vi "Read.vi"(8 "error in (no error)":errorcluster, 9 "Variant":variant, 11 "UDP in":refnum<class "UDP.lvclass">) -> (0 "error out":errorcluster, 2 "String":string, 3 "UDP out":refnum<class "UDP.lvclass">)   [LabVIEW 2013, in "Protocol Classes.lvlib" / "UDP.lvclass"]
uses:
  UDP.lvclass
  Protocol Parent/Methods/Read Parameter.ctl
  UDP.lvclass/UDP.ctl
  Data Access/Read UDP Ref.vi
  Data Access/Write UDP Ref.vi
  Protocol Parent/Protocol Parent.lvclass
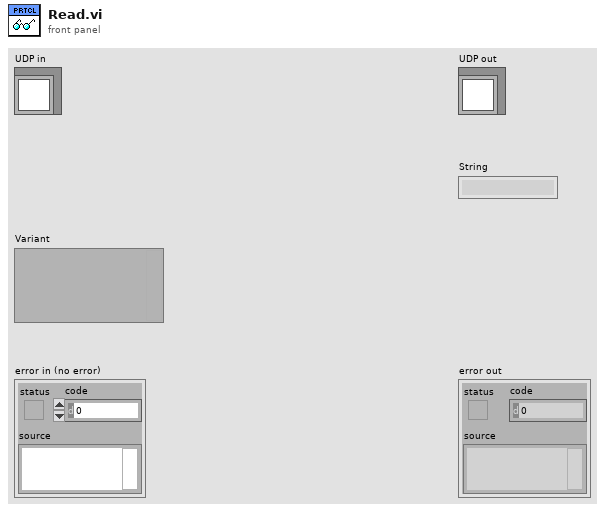
[diagram p1: front panel]
types:
  T1 = typedef "Protocol Classes.lvlib/Protocol Parent.lvclass/Read Parameter.ctl" = cluster{"Wait Type":enum16{"Byte Count", "Wait sec"}, "Wait Value":dbl}
  T2 = enum16{"Standard", "Buffered", "CRLF", "Immediate"}
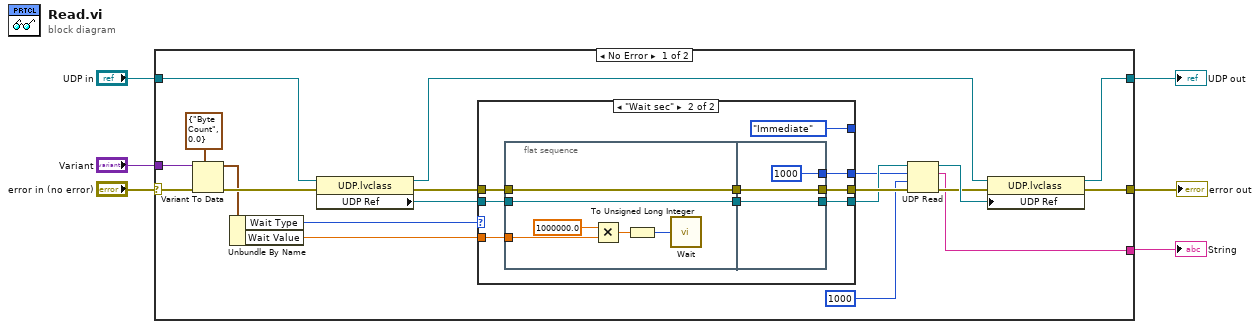
[diagram p0: block diagram]
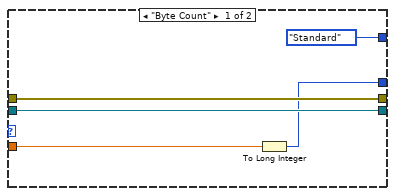
[diagram p2: hidden frame]
diagram:
  n1 = case shown="No Error" "error in (no error)" {
    selector: "error in (no error)" -> [w20 w51]
    tunnel: "UDP in" -> [w26 w50]
    tunnel: [w23 w51] -> w3
    tunnel: [w21 w50] -> w1
    tunnel: "Variant" -> [w18 _]
    tunnel: [w11 _] -> w2
    frame No Error {
      n2 = Variant To Data(error in=w20, type=T1 {"Wait Type"=enum."Byte Count", "Wait Value"=0.0} ("Read Parameter"), Variant=w18) -> (data=w17:T1, error out=w19:errorcluster)
      n3 = Unbundle By Name(w17) -> ("Wait Type"=w13:enum16{"Byte Count", "Wait sec"}, "Wait Value"=w12:dbl)
      n4 = property class="UDP.lvclass"(reference=w26, error in=w19) -> (reference out=w22:refnum<class "UDP.lvclass">, error out=w16:errorcluster, "UDP Ref"=w15:refnum<k16>)
      n5 = case shown="\"Wait sec\"" w13 {
        tunnel: w16 -> [w31 w40]
        tunnel: w15 -> [w29 w39]
        tunnel: [w31 w38] -> w14
        tunnel: [w29 w37] -> w8
        tunnel: [w27 w33] -> w7
        tunnel: w12 -> [w30 w34]
        tunnel: [T2."Standard" ("mode (standard)") T2."Immediate" ("mode (standard)")] -> _
        frame "Byte Count" {
          n6 = To Long Integer(number=w30) -> (32bit integer=w27:i32)
        }
        frame "Wait sec" {
          n7 = flat-sequence {
            tunnel: w39 -> [w45]
            tunnel: w40 -> [w46]
            tunnel: [w46] -> w36
            tunnel: [w45] -> w35
            tunnel: w34 -> [w44]
            tunnel: [w49] -> w38
            tunnel: [w48] -> w37
            tunnel: w36 -> [w49]
            tunnel: w35 -> [w48]
            tunnel: [1000 ("Wait Value")] -> w33
            frame #0 {
              n8 = Multiply(x=1000000.0, y=w44) -> (x*y=w43:dbl)
              n9 = To Unsigned Long Integer(number=w43) -> (unsigned 32bit integer=w41:u32)
              n10 = call "Wait"("Count(uSec)"=w41) -> ()  [unwired: 1 out]
            }
            frame #1 {
            }
          }
        }
      }
      n11 = UDP Read(connection ID=w8, max size (548)=w7, timeout ms (25000)=1000, 8:w14) -> (data out=w11:string, error out=w24:errorcluster, 3:w25:refnum<k16>)  [unwired: 2 out]
      n12 = property class="UDP.lvclass"(reference=w22, error in=w24, "UDP Ref"=w25) -> (reference out=w21:refnum<class "UDP.lvclass">, error out=w23:errorcluster)
    }
    frame Error {
    }
  }
  "error out" <- w3
  "UDP out" <- w1
  "String" <- w2
